vi "Merge Error Wire.vi"(4 "MultiErrors in":refnum<class "MultiErrors.lvclass">, 5 "error in (no error)":errorcluster, 6 "Call Chain (F)":bool) -> (7 "MultiErrors out":refnum<class "MultiErrors.lvclass">)   [LabVIEW 2020, in "VolatusErrorUtilities.lvlib" / "MultiErrors.lvclass"]
uses:
  MultiErrors.lvclass
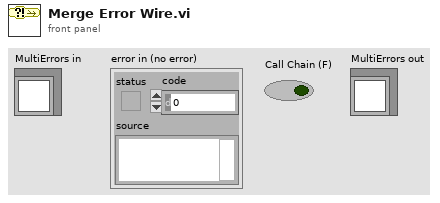
[diagram p1: front panel]
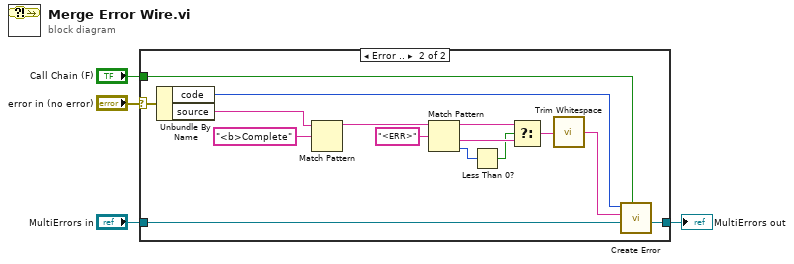
[diagram p0: block diagram]
diagram:
  n1 = case shown="Error .." "error in (no error)" {
    selector: "error in (no error)" -> [_ w19]
    tunnel: "MultiErrors in" -> [w5 w17]
    tunnel: "Call Chain (F)" -> [_ w20]
    tunnel: [w5 w16] -> w1
    frame No Error {
    }
    frame Error {
      n2 = Unbundle By Name(w19) -> ("code"=w18:i32, "source"=w15:string)
      n3 = Match Pattern(string=w15, regular expression="<b>Complete") -> (before substring=w12:string)  [unwired: 1 in, 3 out]
      n4 = Match Pattern(string=w12, regular expression="<ERR>") -> (before substring=w9:string, after substring=w8:string, offset past match=w10:i32)  [unwired: 1 in, 1 out]
      n5 = Less Than 0?(x=w10) -> (x < 0?=w7:bool)
      n6 = Select(t=w9, s=w7, f=w8) -> (s? t:f=w6:string)
      n7 = call <vilib>:"Trim Whitespace.vi"("string"=w6) -> ("trimmed string"=w13:string)  [unwired: 1 in]
      n8 = call "Create Error.vi"("Call Chain (F)"=w20, "MultiErrors in"=w17, "Message"=w13, "Code"=w18) -> ("MultiErrors out"=w16:refnum<class "MultiErrors.lvclass">)  [unwired: 7 in]
    }
  }
  "MultiErrors out" <- w1
